vi "Flash Drive Warning.vi"() -> ()   [LabVIEW 2018]
panel:
  in  "Tab Control":enum32{"warning", "flash drive present"}(tab)
  in  "Test For Drive":bool
  in  "OK":bool
  # "*WARNING*"
  # "No flash drive was detected.  In order to save data during a test a flash drive, formatted as fat32, will need to be plugged into the usb port on the CompactRIO.\n\nPlug in your flash drive and press the Test button below.  Or if you have no plans to save data then press the Continue button."
  # "FLASH DRIVE DETECTED!"
  # "Test data will be saved to this drive.  Press Continue."
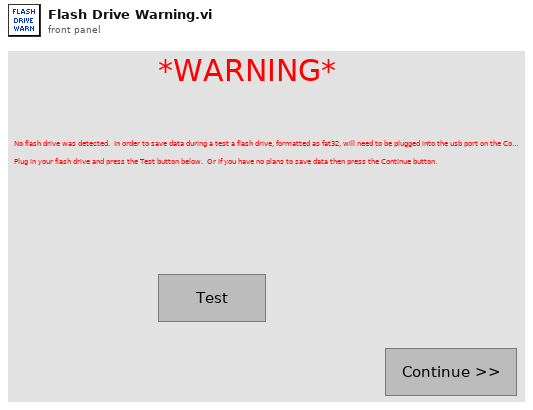
[diagram p1: front panel]
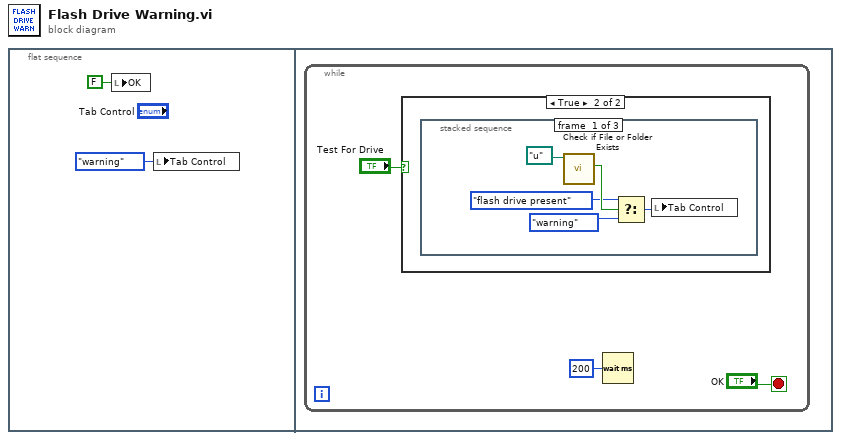
[diagram p0: block diagram]
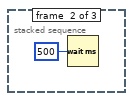
[diagram p3: hidden frame]
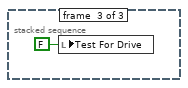
[diagram p4: hidden frame]
diagram:
  n1 = flat-sequence {
    frame #0 {
      n2 = local write "OK"(FALSE ("OK")) -> ()
      n3 = local write "Tab Control"(enum32{"warning", "flash drive present"}."warning" ("Tab Control")) -> ()
    }
    frame #1 {
      n4 = while {
        stop <- "OK" stop-if-true
        n5 = case shown="True" "Test For Drive" {
          frame False {
          }
          frame True {
            n6 = stacked-sequence {
              frame #0 {
                n7 = call <vilib>:"Check if File or Folder Exists.vi"("path"=path "u:/" ("file path (use dialog)")) -> ("file or folder exists?"=w9:bool)  [unwired: 8 in, 2 out]
                n8 = Select(t=enum32{"warning", "flash drive present"}."flash drive present" ("Tab Control"), s=w9, f=enum32{"warning", "flash drive present"}."warning" ("Tab Control")) -> (s? t:f=w6:enum32{"warning", "flash drive present"})
                n9 = local write "Tab Control"(w6) -> ()
              }
              frame #1 {
                n10 = Wait (ms)(milliseconds to wait=u32 500) -> ()  [unwired: 1 out]
              }
              frame #2 {
                n11 = local write "Test For Drive"(FALSE ("Test For Drive")) -> ()
              }
            }
          }
        }
        n12 = Wait (ms)(milliseconds to wait=u32 200) -> ()  [unwired: 1 out]
      }
    }
  }
